vi "Test-Number Count Down.vi"() -> ()   [LabVIEW 2017]
uses:
  user.lib/NEVSTOP-Programming-Palette/Signal/_Instance/_Number Count Down(Array).vi
  user.lib/NEVSTOP-Programming-Palette/Signal/_Instance/_Number Count Down(Element).vi
  user.lib/NEVSTOP-Programming-Palette/Signal/_Instance/_Number Count Down(Array).vi/9de0e42d-c65c-4cbc-a92d-661ac054e2ac.vi
panel:
  in  "Numeric 3":i32[](array[numeric])=[16, 15]
  in  "Numeric 2":i32=15
  in  "Numeric 1":i32=16
  in  "threasholds":i64=1000
  out "left 3":i64[](array[numeric])
  out "left 1":i64
  out "left 2":i64
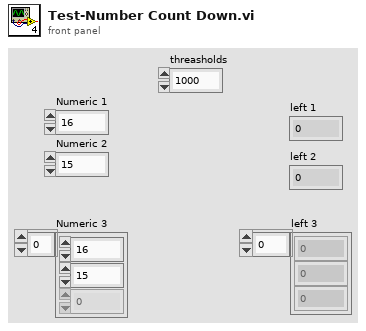
[diagram p1: front panel]
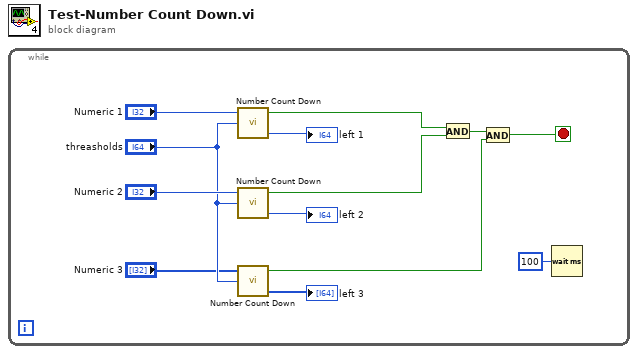
[diagram p0: block diagram]
diagram:
  n1 = while {
    stop <- w3 stop-if-true
    n2 = call-poly "Number Count Down.vi"("number"="Numeric 1", "threashold"="threasholds") -> ("reach?"=w11:bool, "left"=→"left 1":i64)  [unwired: 6 in]
    n3 = call-poly "Number Count Down.vi"("number"="Numeric 2", "threashold"="threasholds") -> ("reach?"=w10:bool, "left"=→"left 2":i64)  [unwired: 6 in]
    n4 = call-poly "Number Count Down.vi"("fixed size array"="Numeric 3", "threashold"="threasholds") -> ("reach?"=w1:bool, "left"=→"left 3":i64[])  [unwired: 6 in]
    n5 = And(x=w11, y=w10) -> (x .and. y?=w2:bool)
    n6 = And(x=w2, y=w1) -> (x .and. y?=w3:bool)
    n7 = Wait (ms)(milliseconds to wait=u32 100) -> ()  [unwired: 1 out]
  }
